vi "Get Policy Details.vi"(8 "error in (no error)":errorcluster, 10 "Name":string, 11 "IoT Session in":refnum<class "IoT Session.lvclass">) -> (0 "error out":errorcluster, 2 "Details":T1, 3 "IoT Session out":refnum<class "IoT Session.lvclass">)   [LabVIEW 2015, in "NI_AWS_IoT.lvlib" / "IoT Session.lvclass"]
uses:
  IoT Session.lvclass
  Policy.ctl
  Core/HTTP Request/Request Options.ctl
  Core/HTTP Request/Name Value Pair.ctl
  Core/HTTP Request/Region handling.ctl
  Core/HTTP Request/URL formatting.ctl
  Core/HTTP Request/HTTP Request.lvclass
  JSON Parsing/NI_JSON Parsing.lvlib
  NI_AWS_IoT.lvlib
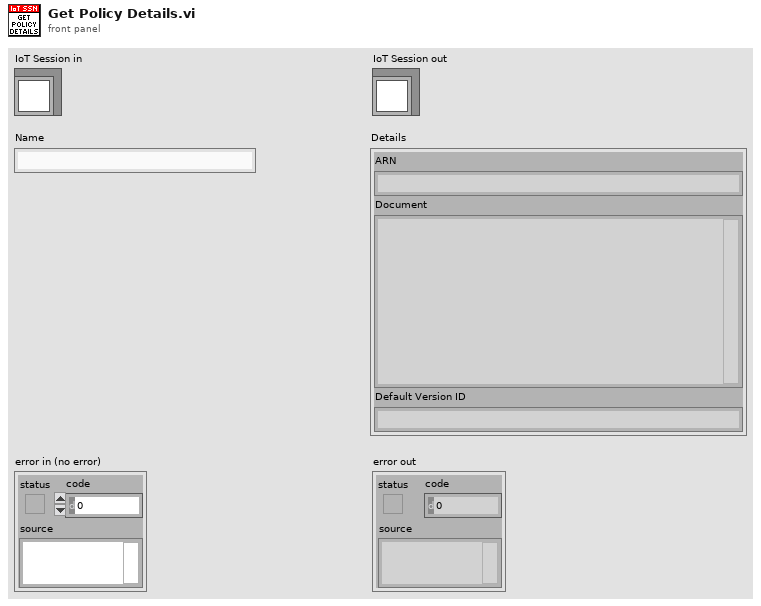
[diagram p1: front panel]
types:
  T1 = typedef "NI_AWS_IoT.lvlib/Policy.ctl" = cluster{"ARN":string, "Document":string, "Default Version ID":string}
  T2 = typedef "NI_AWS_Core.lvlib/HTTP Request.lvclass/Name Value Pair.ctl" = cluster{"name":string, "value":string}
  T3 = typedef "NI_AWS_Core.lvlib/HTTP Request.lvclass/Request Options.ctl" = cluster{"request headers":T2[], "request parameters":T2[], "request body":string, "region handling":T4, "URL formatting":T5}
  T4 = typedef "NI_AWS_Core.lvlib/HTTP Request.lvclass/Region handling.ctl" = enum16{"use region everywhere", "use region (authentication only)", "use region (URL only)", "ignore region everwhere"}
  T5 = typedef "NI_AWS_Core.lvlib/HTTP Request.lvclass/URL formatting.ctl" = enum16{"region-", "region."}
  T6 = typedef "NI_AWS_Core.lvlib/HTTP Request.lvclass/Response.ctl" = cluster{"Headers":string, "Body":string}
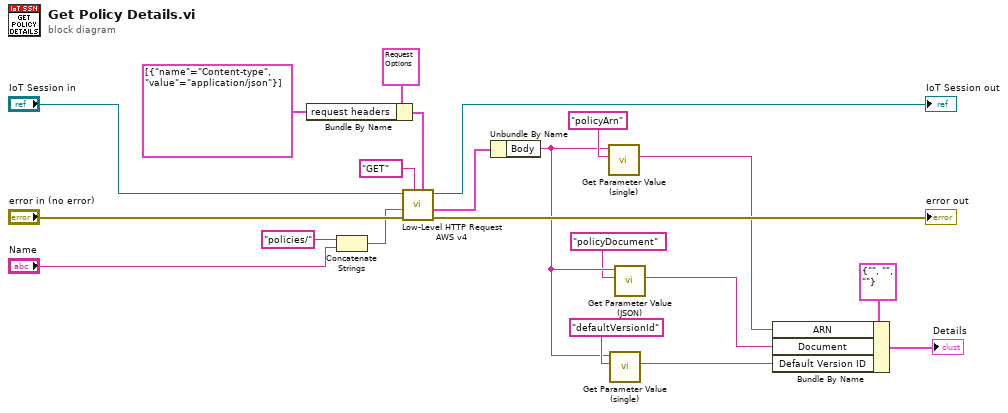
[diagram p0: block diagram]
diagram:
  n1 = Bundle By Name(cluster=T3 {"request headers"=[], "request parameters"=[], "request body"="", "region handling"=enum."use region everywhere", "URL formatting"=enum."region."} ("Request Options"), "request headers"=T2[] [{"name"="Content-type", "value"="application/json"}]) -> (w15:T3)
  n2 = Concatenate Strings("policies/" ("string"), "Name") -> (w10:string)
  n3 = call "Low-Level HTTP Request AWS v4.vi"("Request Options"=w15, "HTTP-Verb"="GET", "error in (no error)"="error in (no error)", "URL Suffix"=w10, "AWS Core in"="IoT Session in") -> ("error out"=→"error out":errorcluster, "Response"=w13:T6, "AWS Core out"=→"IoT Session out":refnum<class "IoT Session.lvclass">)  [unwired: 3 in, 1 out]
  n4 = Unbundle By Name(w13) -> ("Body"=w3:string)
  n5 = call "Get Parameter Value (single).vi"("Parameter Name"="policyArn", "JSON"=w3) -> ("Parameter Value"=w6:string)  [unwired: 6 in, 3 out]
  n6 = call "Get Parameter Value (single).vi"("Parameter Name"="defaultVersionId", "JSON"=w3) -> ("Parameter Value"=w4:string)  [unwired: 6 in, 3 out]
  n7 = call "Get Parameter Value (JSON).vi"("Parameter Name"="policyDocument", "JSON"=w3) -> ("Parameter Value"=w1:string)  [unwired: 6 in, 3 out]
  n8 = Bundle By Name(cluster=T1 {"ARN"="", "Document"="", "Default Version ID"=""} ("Details"), "ARN"=w6, "Document"=w1, "Default Version ID"=w4) -> (→"Details":T1)
